vi "16路数字量输出.vi"(8 "第几组数据":u8, 9 "CAN端口":u16) -> (2 "成功?":bool)   [LabVIEW 2010]
panel:
  # "从1开始"
  # "从0开始"
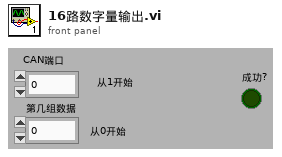
[diagram p1: front panel]
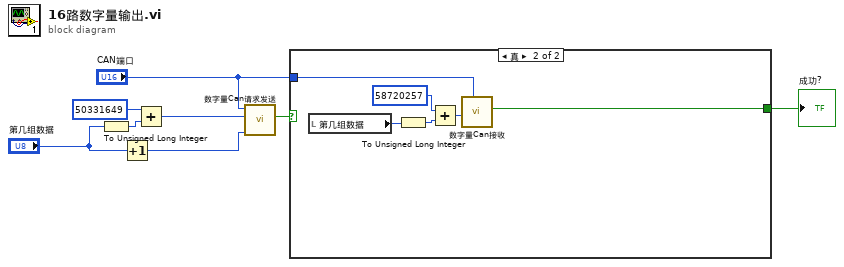
[diagram p0: block diagram]
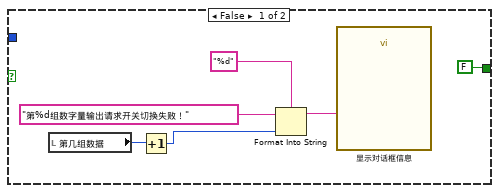
[diagram p2: hidden frame]
diagram:
  n1 = To Unsigned Long Integer(number="第几组数据") -> (unsigned 32bit integer=w6:u32)
  n2 = Increment(x="第几组数据") -> (x+1=w1:u8)
  n3 = Add(x=u32 50331649 ("CANPort"), y=w6) -> (x+y=w5:u32)
  n4 = call "数字量Can请求发送.vi"("第几组数据"=w1, "CANID"=w5, "CANPort"="CAN端口") -> ("发送成功?"=w8:bool)  [unwired: 8 in]
  n5 = case shown="真" w8 {
    tunnel: "CAN端口" -> [_ w16]
    tunnel: [FALSE w15] -> w3
    frame False {
      n6 = local read "第几组数据"() -> (w11:u8)
      n7 = Increment(x=w11) -> (x+1=w10:u8)
      n8 = Format Into String(format string="%d", initial string="第%d组数字量输出请求开关切换失败！", w10) -> (resulting string=w12:string)  [unwired: 1 in, 1 out]
      n9 = call "显示对话框信息"("Message"=w12) -> ()  [unwired: 9 in, 2 out]
    }
    frame True {
      n10 = local read "第几组数据"() -> (w18:u8)
      n11 = To Unsigned Long Integer(number=w18) -> (unsigned 32bit integer=w17:u32)
      n12 = Add(x=u32 58720257 ("CANPort"), y=w17) -> (x+y=w19:u32)
      n13 = call "数字量Can接收.vi"("CANPort"=w16, "匹配CANID"=w19) -> ("成功？"=w15:bool)  [unwired: 8 in, 1 out]
    }
  }
  "成功?" <- w3
